vi "SetVIAttribution.vi"(8 "error in (no error)":errorcluster caption="错误输入（无错误）", 11 "VI ref":refnum<vi>) -> (0 "error out":errorcluster caption="错误输出")   [LabVIEW 2018]
doc: "使用该vi来编辑vi的属性信息"
uses:
  Ctr/WindowAction.ctl
  Ctr/Reentry.ctl
  Ctr/Point.ctl
panel:
  in  "VIInformation":bool
  in  "WindowPosition":bool
  in  "WindowSize":bool
  in  "VIApparence":bool
  in  "VIExec":bool
  in  "VI说明":string
  out "源版本":string
  in  "从源代码文件中分离已编译代码":bool caption="Checkbox"
  in  "优先执行系统":T1(ring)
  in  "优先级":T2(ring)
  out "VI路径":string
  out "VI名称":string
  in  "调用时清空显示控件":bool caption="Checkbox"
  in  "调用时挂起":bool caption="Checkbox"
  in  "运行时自动处理菜单":bool caption="Checkbox"
  in  "UseNowPosition":bool
  in  "坐标":T3
  in  "位置":u16(ring) items=["不改变", "居中", "最大化", "最小化", "自定义"]
  in  "调整窗口大小时缩放前面板上的对象":bool caption="Checkbox"
  in  "使用不同分辨率显示器时保持窗口比例":bool caption="Checkbox"
  in  "UseNowSize":bool
  in  "Height":i32 caption="高度"
  in  "Width":i32 caption="宽度"
  in  "高亮显示Enter布尔":bool caption="Checkbox"
  in  "窗口动作":T4
  in  "允许使用默认运行时快捷菜单":bool caption="Checkbox"
  in  "允许最小化窗口":bool caption="Checkbox"
  in  "允许调整窗口大小":bool caption="Checkbox"
  in  "允许关闭窗口":bool caption="Checkbox"
  in  "运行时透明显示窗口":bool caption="Checkbox"
  in  "如之前未打开则在运行后关闭":bool caption="Checkbox"
  in  "调用时显示前面板":bool caption="Checkbox"
  in  "显示连续运行按钮":bool caption="Checkbox"
  in  "显示运行按钮":bool caption="Checkbox"
  in  "显示终止按钮":bool caption="Checkbox"
  in  "运行时显示工具栏":bool caption="Checkbox"
  in  "显示水平滚动条":bool caption="Checkbox"
  in  "显示垂直滚动条":bool caption="Checkbox"
  in  "显示菜单栏":bool caption="Checkbox"
  in  "窗口包括标题栏":bool caption="Checkbox"
  in  "打开时运行":bool caption="Checkbox"
  in  "启用自动错误处理":bool caption="Checkbox"
  in  "重入":T5 caption="Checkbox"
  in  "在调用vi中内嵌子vi":bool caption="Checkbox"
  in  "允许调试":bool caption="Checkbox"
  in  "Transparency":u8 max=100
  # "执行"
  # "窗口外观"
  # "窗口尺寸"
  # "窗口位置"
  # "VI信息"
  # "%"
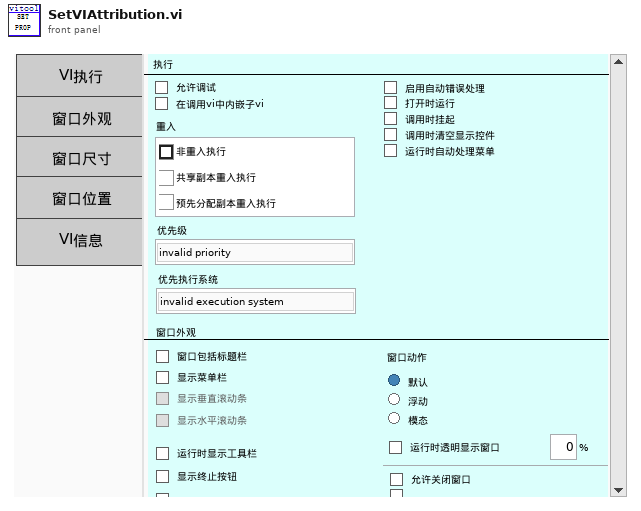
[diagram p1: front panel]
types:
  T1 = enum32{"invalid execution system", "user interface", "standard", "instrument i/o", "data acquisition", "other 1", "other 2", "same as caller"}
  T2 = enum32{"invalid priority", "background priority", "normal priority", "above normal priority", "high priority", "time critical priority", "subroutine"}
  T3 = typedef "Point.ctl" = cluster{"left":dbl, "Top":dbl}
  T4 = typedef "WindowAction.ctl" = enum32{"Default", "Float", "Modal"}
  T5 = typedef "Reentry.ctl" = enum32{"非重入执行", "共享副本重入执行", "预先分配副本重入执行"}
  T6 = enum32{"Bad", "Idle", "Run top level", "Running"}
  T7 = enum16{"Share clones between instances", "Preallocate clone for each instance"}
  T8 = enum32{"Invalid", "Default", "Floating", "Floating/Auto-Hide", "Modal"}
  T9 = enum16{"Always On", "Always Off", "Off While Running"}
  T10 = enum8{"Enabled", "Disabled", "Disabled and Grayed Out"}
  T11 = enum16{"No Scaling", "Scale All Objects", "Scale Single Object"}
  T12 = typedef "LVRectTypeDef.ctl" = cluster{"Left":i16, "Top":i16, "Right":i16, "Bottom":i16}
  T13 = typedef "LVPositionTypeDef.ctl" = cluster{"Left":i32, "Top":i32}
  T14 = typedef "LVBoundsTypeDef.ctl" = cluster{"Width":u32, "Height":u32}
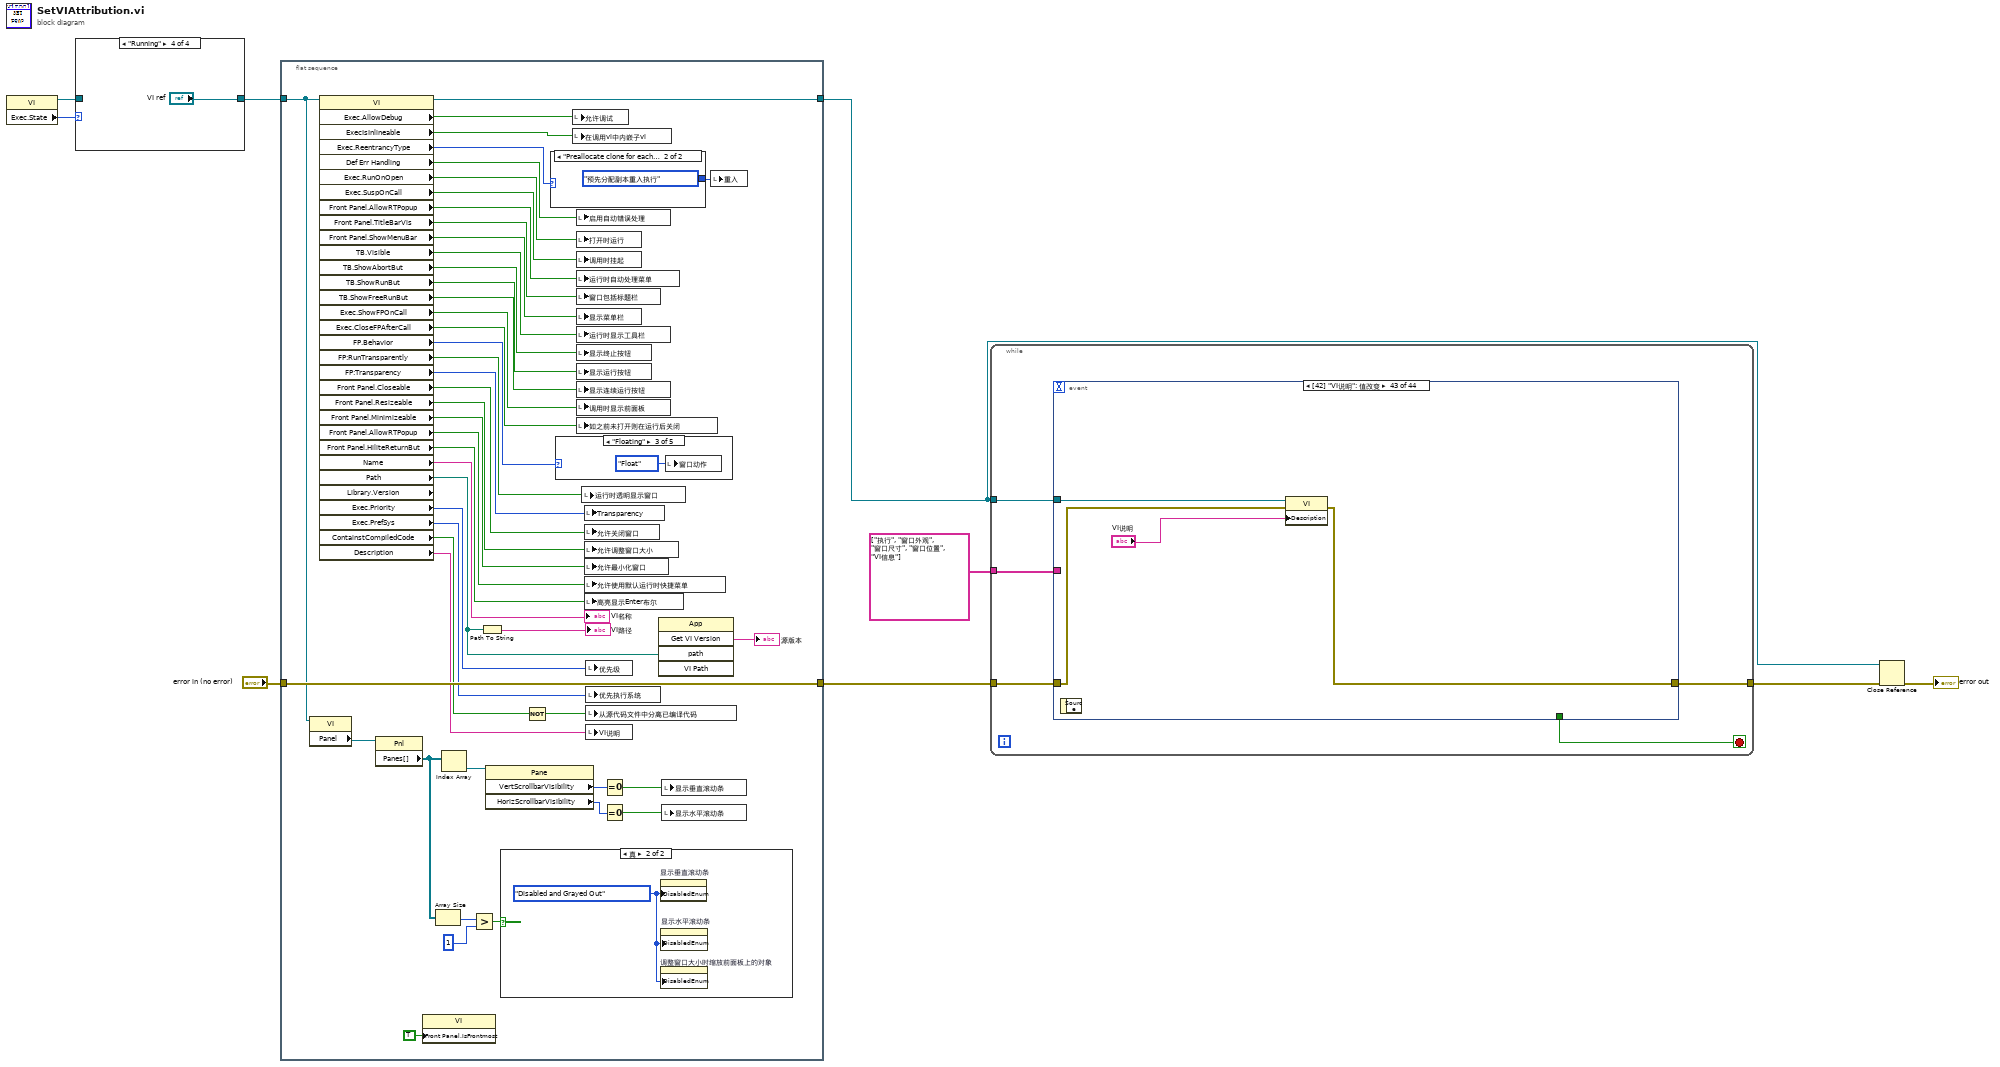
[diagram p0: block diagram]
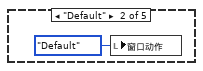
[diagram p7: hidden frame]
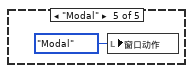
[diagram p9: hidden frame]
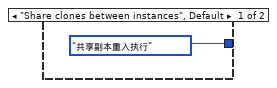
[diagram p10: hidden frame]
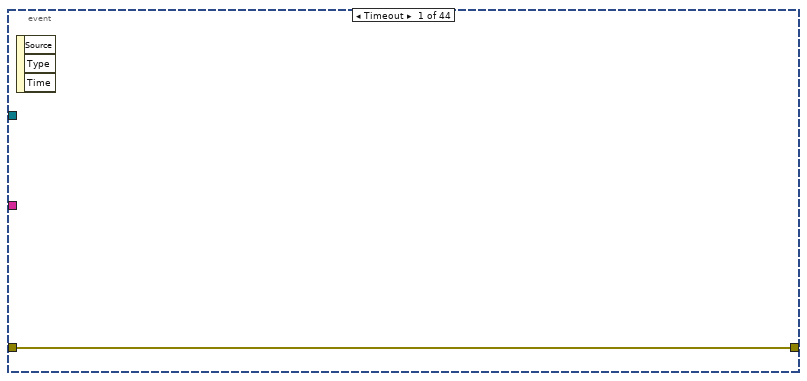
[diagram p11: hidden frame]
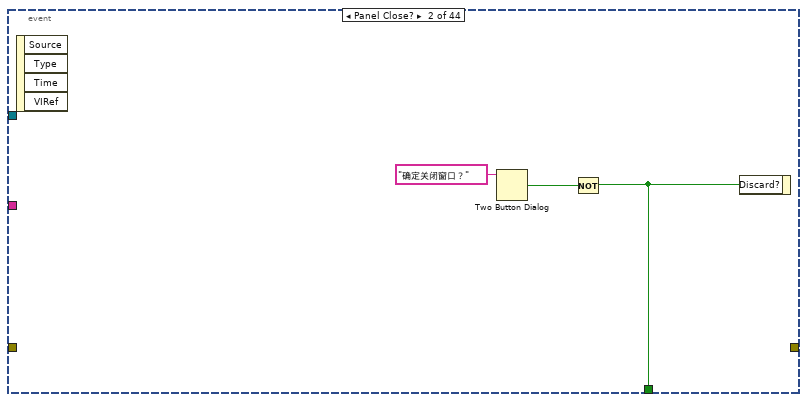
[diagram p12: hidden frame]
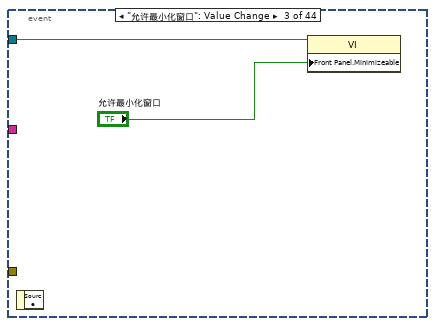
[diagram p13: hidden frame]
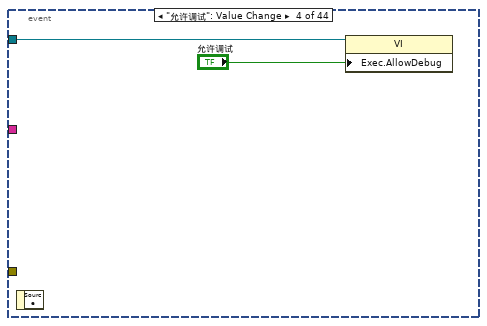
[diagram p14: hidden frame]
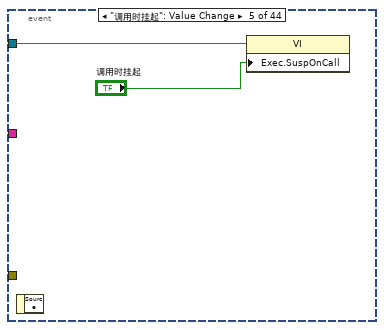
[diagram p15: hidden frame]
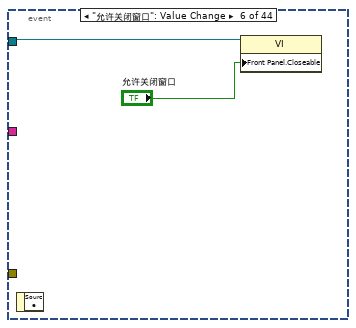
[diagram p16: hidden frame]
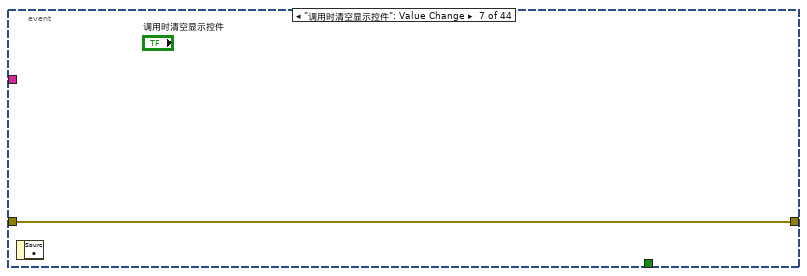
[diagram p17: hidden frame]
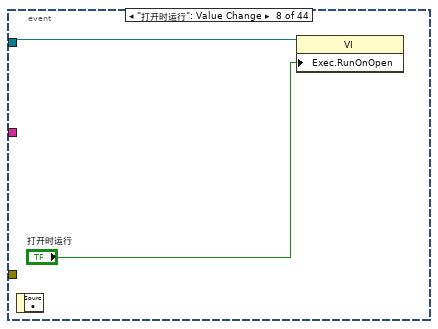
[diagram p18: hidden frame]
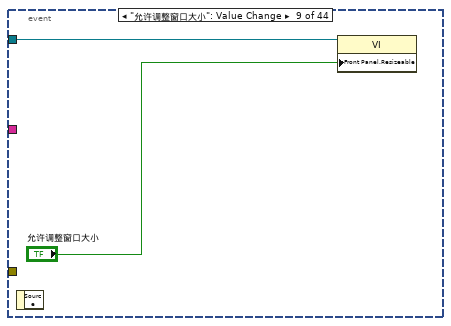
[diagram p19: hidden frame]
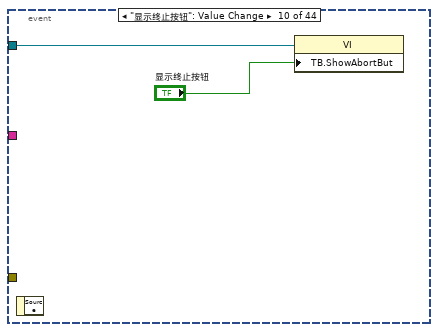
[diagram p20: hidden frame]
diagram:
  n1 = property class="VI"() -> (reference out=w5:refnum<vi>, "Exec.State"=w6:T6)  [unwired: 2 in, 1 out]
  n2 = case shown="\"Running\"" w6 {
    tunnel: [w10 w11 w12 "VI ref"] -> w9
    tunnel: w5 -> [w10 w11 w12 _]
    frame "Bad", Default {
    }
    frame "Idle" {
    }
    frame "Run top level" {
    }
    frame "Running" {
    }
  }
  n3 = flat-sequence {
    tunnel: w9 -> [w16]
    tunnel: [w60] -> w2
    tunnel: "error in (no error)" -> [w59]
    tunnel: [w59] -> w7
    frame #0 {
      n4 = property class="VI"(reference=w16) -> ("Panel"=w48:refnum<vi>)  [unwired: 1 in, 2 out]
      n5 = property class="VI" props=["Exec.AllowDebug", "ExecIsInlineable", "Exec.ReentrancyType", "Def Err Handling", "Exec.RunOnOpen", "Exec.SuspOnCall", "Front Panel.AllowRTPopup", "Front Panel.TitleBarVis", "Front Panel.ShowMenuBar", "TB.Visible", "TB.ShowAbortBut", "TB.ShowRunBut", "TB.ShowFreeRunBut", "Exec.ShowFPOnCall", "Exec.CloseFPAfterCall", "FP.Behavior", "FP:RunTransparently", "FP:Transparency", "Front Panel.Closeable", "Front Panel.Resizeable", "Front Panel.Minimizeable", "Front Panel.AllowRTPopup", "Front Panel.HiliteReturnBut", "Name", "Path", "Library.Version", "Exec.Priority", "Exec.PrefSys", "ContainstCompiledCode", "Description"](reference=w16) -> (reference out=w60:refnum<vi>, "Exec.AllowDebug"=w58:bool, "ExecIsInlineable"=w57:bool, "Exec.ReentrancyType"=w56:T7, "Def Err Handling"=w54:bool, "Exec.RunOnOpen"=w53:bool, "Exec.SuspOnCall"=w52:bool, "Front Panel.AllowRTPopup"=w51:bool, "Front Panel.TitleBarVis"=w50:bool, "Front Panel.ShowMenuBar"=w49:bool, "TB.Visible"=w42:bool, "TB.ShowAbortBut"=w41:bool, "TB.ShowRunBut"=w40:bool, "TB.ShowFreeRunBut"=w39:bool, "Exec.ShowFPOnCall"=w38:bool, "Exec.CloseFPAfterCall"=w37:bool, "FP.Behavior"=w36:T8, "FP:RunTransparently"=w35:bool, "FP:Transparency"=w34:u8, "Front Panel.Closeable"=w33:bool, "Front Panel.Resizeable"=w32:bool, "Front Panel.Minimizeable"=w31:bool, "Front Panel.AllowRTPopup"=w30:bool, "Front Panel.HiliteReturnBut"=w29:bool, "Name"=→"VI名称":string, "Path"=w15:path, "Exec.Priority"=w26:T2, "Exec.PrefSys"=w25:T1, "ContainstCompiledCode"=w20:bool, "Description"=w17:string)  [unwired: 1 in, 2 out]
      n6 = property class="Pnl"(reference=w48) -> ("Panes[]"=w24:refnum<vi>[])  [unwired: 1 in, 2 out]
      n7 = property class="VI"("Front Panel.IsFrontmost"=TRUE ("前面板窗口:在最前")) -> ()  [unwired: 2 in, 2 out]
      n8 = Array Size(array=w24) -> (size(s)=w23:i32)
      n9 = Index Array(array=w24) -> (element=w47:refnum<vi>)  [unwired: 1 in]
      n10 = Greater?(x=w23, y=1) -> (0:w21:bool)
      n11 = Path To String(path=w15) -> (string=→"VI路径":string)
      n12 = property class="Pane"(reference=w47) -> ("VertScrollbarVisibility"=w46:T9, "HorizScrollbarVisibility"=w44:T9)  [unwired: 1 in, 2 out]
      n13 = case shown="真" w21 {
        frame False {
        }
        frame True {
          w61 = T10."Disabled and Grayed Out" ("禁用")
          n14 = property on="显示垂直滚动条" class="Bool (严格)"("DisabledEnum"=w61) -> ()  [unwired: 2 in, 2 out]
          n15 = property on="显示水平滚动条" class="Bool (严格)"("DisabledEnum"=w61) -> ()  [unwired: 2 in, 2 out]
          n16 = property on="调整窗口大小时缩放前面板上的对象" class="Bool (严格)"("DisabledEnum"=w61) -> ()  [unwired: 2 in, 2 out]
        }
      }
      n17 = Not(x=w20) -> (.not. x?=w19:bool)
      n18 = case shown="\"Preallocate clone for each instance\"" w56 {
        tunnel: [Reentry."共享副本重入执行" ("重入") Reentry."预先分配副本重入执行" ("重入")] -> w55
        frame "Share clones between instances", Default {
        }
        frame "Preallocate clone for each instance" {
        }
      }
      n19 = case shown="\"Floating\"" w36 {
        frame "Invalid", Default {
        }
        frame "Default" {
          n20 = local write "窗口动作"(WindowAction."Default" ("窗口动作")) -> ()
        }
        frame "Floating" {
          n21 = local write "窗口动作"(WindowAction."Float" ("窗口动作")) -> ()
        }
        frame "Floating/Auto-Hide" {
        }
        frame "Modal" {
          n22 = local write "窗口动作"(WindowAction."Modal" ("窗口动作")) -> ()
        }
      }
      n23 = local write "允许调试"(w58) -> ()
      n24 = local write "在调用vi中内嵌子vi"(w57) -> ()
      n25 = local write "启用自动错误处理"(w54) -> ()
      n26 = local write "打开时运行"(w53) -> ()
      n27 = local write "调用时挂起"(w52) -> ()
      n28 = local write "运行时自动处理菜单"(w51) -> ()
      n29 = local write "窗口包括标题栏"(w50) -> ()
      n30 = local write "显示菜单栏"(w49) -> ()
      n31 = local write "运行时显示工具栏"(w42) -> ()
      n32 = local write "显示终止按钮"(w41) -> ()
      n33 = local write "显示运行按钮"(w40) -> ()
      n34 = local write "显示连续运行按钮"(w39) -> ()
      n35 = local write "调用时显示前面板"(w38) -> ()
      n36 = local write "如之前未打开则在运行后关闭"(w37) -> ()
      n37 = local write "运行时透明显示窗口"(w35) -> ()
      n38 = local write "Transparency"(w34) -> ()
      n39 = local write "允许关闭窗口"(w33) -> ()
      n40 = local write "允许调整窗口大小"(w32) -> ()
      n41 = local write "允许最小化窗口"(w31) -> ()
      n42 = local write "允许使用默认运行时快捷菜单"(w30) -> ()
      n43 = local write "高亮显示Enter布尔"(w29) -> ()
      n44 = local write "优先级"(w26) -> ()
      n45 = local write "优先执行系统"(w25) -> ()
      n46 = local write "从源代码文件中分离已编译代码"(w19) -> ()
      n47 = local write "VI说明"(w17) -> ()
      n48 = Equal To 0?(x=w46) -> (x = 0?=w45:bool)
      n49 = Equal To 0?(x=w44) -> (x = 0?=w43:bool)
      n50 = invoke class="App" method="Get VI Version"("path"=w15) -> ("GetVIVers"=→"源版本":string)  [unwired: 4 in, 4 out]
      n51 = local write "显示垂直滚动条"(w45) -> ()
      n52 = local write "显示水平滚动条"(w43) -> ()
      n53 = local write "重入"(w55) -> ()
    }
  }
  n54 = while {
    tunnel: w2 -> [w70]
    tunnel: w7 -> [w69]
    tunnel: [w68] -> w3
    tunnel: string[] ["执行", "窗口外观", "窗口尺寸", "窗口位置", "VI信息"] -> [w67]
    stop <- w71 stop-if-true
    n55 = event shown="[42] \"VI说明\": 值改变" {
      selector: _ -> [_ _ _ _ _ _ _ _ _ _ _ _ _ _ _ _ _ _ _ _ _ _ _ _ _ _ _ _ _ _ _ _ _ _ _ _ _ _ _ _ _ _ _ _]
      dyn-events: _ -> [_ _ _ _ _ _ _ _ _ _ _ _ _ _ _ _ _ _ _ _ _ _ _ _ _ _ _ _ _ _ _ _ _ _ _ _ _ _ _ _ _ _ _ _]
      timeout: _ -> [_ _ _ _ _ _ _ _ _ _ _ _ _ _ _ _ _ _ _ _ _ _ _ _ _ _ _ _ _ _ _ _ _ _ _ _ _ _ _ _ _ _ _ _]
      tunnel: [_ w74 _ _ _ _ _ _ _ _ _ _ _ _ _ _ _ _ _ _ _ _ _ _ _ _ _ _ _ _ _ _ _ _ _ _ _ _ _ _ _ _ _ _] -> w71
      tunnel: w70 -> [_ _ w77 w79 w81 w83 _ w86 w88 w90 w92 w94 w96 w98 w100 w102 w104 w106 w108 w110 w112 w114 w115 w122 w136 _ w144 w147 w156 w161 w169 w179 w183 w189 w198 _ _ _ _ _ w231 w235 w239 w244]
      tunnel: w69 -> [w72 _ _ _ _ _ w84 _ _ _ _ _ _ _ _ _ _ _ _ _ _ _ w117 _ _ _ _ _ w155 w158 _ w178 w181 w185 w195 w204 w213 _ w218 w223 w229 w233 w237 w241]
      tunnel: [w72 _ _ _ _ _ w84 _ _ _ _ _ _ _ _ _ _ _ _ _ _ _ w116 _ _ _ _ _ w151 w157 _ w177 w182 w190 w194 w204 w213 _ w218 w223 w228 w232 w236 w240] -> w68
      tunnel: w67 -> [_ _ _ _ _ _ _ _ _ _ _ _ _ _ _ _ _ _ _ _ _ _ _ _ _ _ _ _ _ _ _ _ _ _ _ w208 w211 w217 w222 w227 _ _ _ _]
      event Timeout {
        n56 = event-data() -> ()  [unwired: 1 in, 3 out]
      }
      event Panel Close? {
        n57 = event-data() -> ()  [unwired: 1 in, 4 out]
        n58 = Two Button Dialog(message="确定关闭窗口？" ("消息")) -> (T button?=w75:bool)  [unwired: 2 in]
        n59 = Not(x=w75) -> (.not. x?=w74:bool)
        n60 = event-data("Discard?"=w74) -> ()  [unwired: 1 in, 1 out]
      }
      event "允许最小化窗口": Value Change {
        n61 = event-data() -> ()  [unwired: 1 in, 1 out]
        n62 = property class="VI"(reference=w77, "Front Panel.Minimizeable"="允许最小化窗口") -> ()  [unwired: 1 in, 2 out]
      }
      event "允许调试": Value Change {
        n63 = event-data() -> ()  [unwired: 1 in, 1 out]
        n64 = property class="VI"(reference=w79, "Exec.AllowDebug"="允许调试") -> ()  [unwired: 1 in, 2 out]
      }
      event "调用时挂起": Value Change {
        n65 = event-data() -> ()  [unwired: 1 in, 1 out]
        n66 = property class="VI"(reference=w81, "Exec.SuspOnCall"="调用时挂起") -> ()  [unwired: 1 in, 2 out]
      }
      event "允许关闭窗口": Value Change {
        n67 = event-data() -> ()  [unwired: 1 in, 1 out]
        n68 = property class="VI"(reference=w83, "Front Panel.Closeable"="允许关闭窗口") -> ()  [unwired: 1 in, 2 out]
      }
      event "调用时清空显示控件": Value Change {
        n69 = event-data() -> ()  [unwired: 1 in, 1 out]
      }
      event "打开时运行": Value Change {
        n70 = event-data() -> ()  [unwired: 1 in, 1 out]
        n71 = property class="VI"(reference=w86, "Exec.RunOnOpen"="打开时运行") -> ()  [unwired: 1 in, 2 out]
      }
      event "允许调整窗口大小": Value Change {
        n72 = event-data() -> ()  [unwired: 1 in, 1 out]
        n73 = property class="VI"(reference=w88, "Front Panel.Resizeable"="允许调整窗口大小") -> ()  [unwired: 1 in, 2 out]
      }
      event "显示终止按钮": Value Change {
        n74 = event-data() -> ()  [unwired: 1 in, 1 out]
        n75 = property class="VI"(reference=w90, "TB.ShowAbortBut"="显示终止按钮") -> ()  [unwired: 1 in, 2 out]
      }
      event "在调用vi中内嵌子vi": Value Change {
        n76 = event-data() -> ()  [unwired: 1 in, 1 out]
        n77 = property class="VI"(reference=w92, "ExecInlining"="在调用vi中内嵌子vi") -> ()  [unwired: 1 in, 2 out]
      }
      event "运行时显示工具栏": Value Change {
        n78 = event-data() -> ()  [unwired: 1 in, 1 out]
        n79 = property class="VI"(reference=w94, "TB.Visible"="运行时显示工具栏") -> ()  [unwired: 1 in, 2 out]
      }
      event "显示运行按钮": Value Change {
        n80 = event-data() -> ()  [unwired: 1 in, 1 out]
        n81 = property class="VI"(reference=w96, "TB.ShowRunBut"="显示运行按钮") -> ()  [unwired: 1 in, 2 out]
      }
      event "显示连续运行按钮": Value Change {
        n82 = event-data() -> ()  [unwired: 1 in, 1 out]
        n83 = property class="VI"(reference=w98, "TB.ShowFreeRunBut"="显示连续运行按钮") -> ()  [unwired: 1 in, 2 out]
      }
      event "显示菜单栏": Value Change {
        n84 = event-data() -> ()  [unwired: 1 in, 1 out]
        n85 = property class="VI"(reference=w100, "Front Panel.ShowMenuBar"="显示菜单栏") -> ()  [unwired: 1 in, 2 out]
      }
      event "窗口包括标题栏": Value Change {
        n86 = event-data() -> ()  [unwired: 1 in, 1 out]
        n87 = property class="VI"(reference=w102, "Front Panel.TitleBarVis"="窗口包括标题栏") -> ()  [unwired: 1 in, 2 out]
      }
      event "调用时显示前面板": Value Change {
        n88 = event-data() -> ()  [unwired: 1 in, 1 out]
        n89 = property class="VI"(reference=w104, "Exec.ShowFPOnCall"="调用时显示前面板") -> ()  [unwired: 1 in, 2 out]
      }
      event "运行时自动处理菜单": Value Change {
        n90 = event-data() -> ()  [unwired: 1 in, 1 out]
        n91 = property class="VI"(reference=w106, "Front Panel.AllowRTPopup"="运行时自动处理菜单") -> ()  [unwired: 1 in, 2 out]
      }
      event "启用自动错误处理": Value Change {
        n92 = event-data() -> ()  [unwired: 1 in, 1 out]
        n93 = property class="VI"(reference=w108, "Def Err Handling"="启用自动错误处理") -> ()  [unwired: 1 in, 2 out]
      }
      event "运行时透明显示窗口": Value Change {
        n94 = event-data() -> ()  [unwired: 1 in, 1 out]
        n95 = property class="VI"(reference=w110, "FP:RunTransparently"="运行时透明显示窗口") -> ()  [unwired: 1 in, 2 out]
      }
      event "Transparency": Value Change {
        n96 = event-data() -> ()  [unwired: 1 in, 1 out]
        n97 = property class="VI"(reference=w112, "FP:Transparency"="Transparency") -> ()  [unwired: 1 in, 2 out]
      }
      event "如之前未打开则在运行后关闭": Value Change {
        n98 = event-data() -> ()  [unwired: 1 in, 1 out]
        n99 = property class="VI"(reference=w114, "Exec.CloseFPAfterCall"="如之前未打开则在运行后关闭") -> ()  [unwired: 1 in, 2 out]
      }
      event "使用不同分辨率显示器时保持窗口比例": Value Change {
        n100 = event-data() -> ()  [unwired: 1 in, 1 out]
        n101 = property class="VI"(reference=w115, error in=w117, "Front Panel.KeepWinProps"="使用不同分辨率显示器时保持窗口比例") -> (error out=w116:errorcluster)  [unwired: 1 out]
      }
      event Value Change {
        n102 = event-data() -> ()  [unwired: 1 in, 1 out]
        n103 = Greater Than 0?(x="重入") -> (x > 0?=w121:bool)
        n104 = property class="VI"(reference=w122, "Exec.IsReentrant"=w121) -> (reference out=w119:refnum<vi>)  [unwired: 1 in, 1 out]
        n105 = case shown="\"预先分配副本重入执行\"" "重入" {
          tunnel: w119 -> [_ w124 w125]
          frame "非重入执行", Default {
          }
          frame "共享副本重入执行" {
            n106 = property class="VI"(reference=w124, "Exec.ReentrancyType"=0) -> ()  [unwired: 1 in, 2 out]
          }
          frame "预先分配副本重入执行" {
            n107 = property class="VI"(reference=w125, "Exec.ReentrancyType"=1) -> ()  [unwired: 1 in, 2 out]
          }
        }
      }
      event "Width", "Height": Value Change {
        n108 = event-data() -> ()  [unwired: 1 in, 1 out]
        n109 = property class="VI"(reference=w136) -> (reference out=w135:refnum<vi>, "Front Panel.WinBounds"=w133:T12)  [unwired: 1 in, 1 out]
        n110 = Unbundle By Name(w133) -> ("Left"=w134:i16, "Top"=w130:i16)
        n111 = Add(x=w134, y="Width") -> (x+y=w131:i32)
        n112 = Add(x=w130, y="Height") -> (x+y=w128:i32)
        n113 = Bundle By Name(cluster=w133, "Right"=w131, "Bottom"=w128) -> (w127:T12)
        n114 = property class="VI"(reference=w135, "Front Panel.WinBounds"=w127) -> ()  [unwired: 1 in, 2 out]
      }
      event "位置": Value Change {
        n115 = event-data() -> ()  [unwired: 1 in, 1 out]
        n116 = Equal?(x="位置", y=u16 4) -> (x = y?=w140:bool)
        n117 = Select(t=T10."Enabled" ("禁用"), s=w140, f=T10."Disabled and Grayed Out") -> (s? t:f=w137:T10)
        n118 = property on="坐标" class="Clust (严格)"("DisabledEnum"=w137) -> ()  [unwired: 2 in, 2 out]
        n119 = property on="UseNowPosition" class="Bool"("DisabledEnum"=w137) -> ()  [unwired: 2 in, 2 out]
      }
      event "高亮显示Enter布尔": Value Change {
        n120 = event-data() -> ()  [unwired: 1 in, 1 out]
        n121 = property class="VI"(reference=w144, "Front Panel.HiliteReturnBut"="高亮显示Enter布尔") -> ()  [unwired: 1 in, 2 out]
      }
      event Value Change {
        n122 = event-data() -> ()  [unwired: 1 in, 1 out]
        n123 = property class="VI"(reference=w147) -> ("Panel"=w146:refnum<vi>)  [unwired: 1 in, 2 out]
        n124 = local read "位置"() -> (w148:u16)
        n125 = case shown="4" w148 {
          tunnel: w146 -> [_ _ w150]
          tunnel: "坐标" -> [_ _ w149]
          frame 0, Default {
          }
          frame 1 {
          }
          frame 4 {
            n126 = property class="Pnl"(reference=w150, "Position"=w149) -> ()  [unwired: 1 in, 2 out]
          }
        }
      }
      event "UseNowPosition": Value Change {
        n127 = event-data() -> ()  [unwired: 1 in, 1 out]
        n128 = property class="VI"(reference=w156, error in=w155) -> (error out=w152:errorcluster, "Panel"=w154:refnum<vi>)  [unwired: 1 out]
        n129 = property class="Pnl"(reference=w154, error in=w152) -> (error out=w151:errorcluster, "Position"=w153:T13)  [unwired: 1 out]
        n130 = local write "坐标"(w153) -> ()
      }
      event Value Change {
        n131 = event-data() -> ()  [unwired: 1 in, 1 out]
        n132 = case shown="\"Float\"" "窗口动作" {
          tunnel: [T8."Default" ("前面板窗口:动作") T8."Floating" ("前面板窗口:动作") T8."Modal" ("前面板窗口:动作")] -> w159
          frame "Default", Default {
          }
          frame "Float" {
          }
          frame "Modal" {
          }
        }
        n133 = property class="VI"(reference=w161, error in=w158, "FP.Behavior"=w159) -> (error out=w157:errorcluster)  [unwired: 1 out]
      }
      event "UseNowSize": Value Change {
        n134 = event-data() -> ()  [unwired: 1 in, 1 out]
        n135 = property class="VI"(reference=w169) -> ("Panel"=w168:refnum<vi>)  [unwired: 1 in, 2 out]
        n136 = property class="Pnl"(reference=w168) -> ("Bounds"=w167:T14)  [unwired: 1 in, 2 out]
        n137 = Unbundle By Name(w167) -> ("Width"=w166:u32, "Height"=w165:u32)
        n138 = local write "Width"(w166) -> ()
        n139 = local write "Height"(w165) -> ()
      }
      event "调整窗口大小时缩放前面板上的对象": Value Change {
        n140 = event-data() -> ()  [unwired: 1 in, 1 out]
        n141 = property class="VI"(reference=w179, error in=w178) -> (error out=w177:errorcluster, "Panel"=w176:refnum<vi>)  [unwired: 1 out]
        n142 = Select(t=T11."Scale All Objects" ("缩放模式"), s="调整窗口大小时缩放前面板上的对象", f=T11."No Scaling") -> (s? t:f=w171:T11)
        n143 = property class="Pnl"(reference=w176) -> ("Panes[]"=w175:refnum<vi>[])  [unwired: 1 in, 2 out]
        n144 = Index Array(array=w175) -> (element=w174:refnum<vi>)  [unwired: 1 in]
        n145 = invoke class="Pane" method="Set Scaling"(reference=w174, "ScalingMode"=w171) -> ()  [unwired: 3 in, 5 out]
      }
      event "允许使用默认运行时快捷菜单": Value Change {
        n146 = event-data() -> ()  [unwired: 1 in, 1 out]
        n147 = property class="VI"(reference=w183, error in=w181, "Front Panel.AllowRTPopup"="允许使用默认运行时快捷菜单") -> (error out=w182:errorcluster)  [unwired: 1 out]
      }
      event "显示垂直滚动条": Value Change {
        n148 = event-data() -> ()  [unwired: 1 in, 1 out]
        n149 = property class="VI"(reference=w189) -> ("Panel"=w188:refnum<vi>)  [unwired: 1 in, 2 out]
        n150 = property class="Pnl"(reference=w188) -> ("Panes[]"=w187:refnum<vi>[])  [unwired: 1 in, 2 out]
        n151 = Select(t=T9."Always On" ("垂直滚动条可见"), s="显示垂直滚动条", f=T9."Always Off" ("垂直滚动条可见")) -> (s? t:f=w184:T9)
        n152 = Index Array(array=w187) -> (element=w186:refnum<vi>)  [unwired: 1 in]
        n153 = property on="属性节点" class="Pane"(reference=w186, error in=w185, "VertScrollbarVisibility"=w184) -> (error out=w190:errorcluster)  [unwired: 1 out]
      }
      event "显示水平滚动条": Value Change {
        n154 = event-data() -> ()  [unwired: 1 in, 1 out]
        n155 = property class="VI"(reference=w198) -> ("Panel"=w200:refnum<vi>)  [unwired: 1 in, 2 out]
        n156 = property class="Pnl"(reference=w200) -> ("Panes[]"=w199:refnum<vi>[])  [unwired: 1 in, 2 out]
        n157 = Select(t=T9."Always On" ("水平滚动条可见"), s="显示水平滚动条", f=T9."Always Off") -> (s? t:f=w196:T9)
        n158 = Index Array(array=w199) -> (element=w197:refnum<vi>)  [unwired: 1 in]
        n159 = property class="Pane"(reference=w197, error in=w195, "HorizScrollbarVisibility"=w196) -> (error out=w194:errorcluster)  [unwired: 1 out]
      }
      event "VIExec": Value Change {
        n160 = event-data() -> ()  [unwired: 1 in, 1 out]
        n161 = control-ref of="本VI"() -> (w206:refnum<vi>)
        n162 = Index Array(array=w208, index=0 ("索引")) -> (element=w205:string)
        n163 = call "MoveScroll.vi"("Text"=w205, "VI输入"=w206) -> ()  [unwired: 10 in]
      }
      event "VIApparence": Value Change {
        n164 = event-data() -> ()  [unwired: 1 in, 1 out]
        n165 = control-ref of="本VI"() -> (w212:refnum<vi>)
        n166 = Index Array(array=w211, index=1 ("索引")) -> (element=w209:string)
        n167 = call "MoveScroll.vi"("Text"=w209, "VI输入"=w212) -> ()  [unwired: 10 in]
      }
      event "WindowSize": Value Change {
        n168 = event-data() -> ()  [unwired: 1 in, 1 out]
        n169 = control-ref of="本VI"() -> (w214:refnum<vi>)
        n170 = Index Array(array=w217, index=2 ("索引")) -> (element=w215:string)
        n171 = call "MoveScroll.vi"("Text"=w215, "VI输入"=w214) -> ()  [unwired: 10 in]
      }
      event "WindowPosition": Value Change {
        n172 = event-data() -> ()  [unwired: 1 in, 1 out]
        n173 = Index Array(array=w222, index=3 ("索引")) -> (element=w220:string)
        n174 = control-ref of="本VI"() -> (w219:refnum<vi>)
        n175 = call "MoveScroll.vi"("Text"=w220, "VI输入"=w219) -> ()  [unwired: 10 in]
      }
      event "VIInformation": Value Change {
        n176 = event-data() -> ()  [unwired: 1 in, 1 out]
        n177 = Index Array(array=w227, index=4 ("索引")) -> (element=w225:string)
        n178 = control-ref of="本VI"() -> (w224:refnum<vi>)
        n179 = call "MoveScroll.vi"("Text"=w225, "VI输入"=w224) -> ()  [unwired: 10 in]
      }
      event "优先执行系统": Value Change {
        n180 = event-data() -> ()  [unwired: 1 in, 1 out]
        n181 = property class="VI"(reference=w231, error in=w229, "Exec.PrefSys"="优先执行系统") -> (error out=w228:errorcluster)  [unwired: 1 out]
      }
      event "优先级": Value Change {
        n182 = event-data() -> ()  [unwired: 1 in, 1 out]
        n183 = property class="VI"(reference=w235, error in=w233, "Exec.Priority"="优先级") -> (error out=w232:errorcluster)  [unwired: 1 out]
      }
      event "VI说明": Value Change {
        n184 = event-data() -> ()  [unwired: 1 in, 1 out]
        n185 = property class="VI"(reference=w239, error in=w237, "Description"="VI说明") -> (error out=w236:errorcluster)  [unwired: 1 out]
      }
      event "从源代码文件中分离已编译代码": Value Change {
        n186 = event-data() -> ()  [unwired: 1 in, 1 out]
        n187 = Not(x="从源代码文件中分离已编译代码") -> (.not. x?=w242:bool)
        n188 = property class="VI"(reference=w244, error in=w241, "ContainstCompiledCode"=w242) -> (error out=w240:errorcluster)  [unwired: 1 out]
      }
    }
  }
  n189 = Close Reference(reference=w2, error in (no error)=w3) -> (error out=→"error out":errorcluster)
